vi "Speed Control 1 - Just before second motor.vi"(11 "queue in":refnum<queue>) -> ()   [LabVIEW 2014]
uses:
  controls/UI Data.ctl
  controls/Control ConfigurationSam.ctl
  controls/EncoderController.ctl
  <vilib>/Platform/TimedLoop/XDataNode/timing_clust.ctl
  <vilib>/Platform/TimedLoop/XDataNode/nitl_modes.ctl
  <vilib>/Platform/TimedLoop/XDataNode/wakeup.ctl
  controls/Control StateSam.ctl
  <vilib>/Platform/TimedLoop/XDataNode/loadnilvce.vi
  <vilib>/addons/control/pid/pid.llb/PID (DBL).vi
  <vilib>/addons/control/pid/pid.llb/PID Percentage to EGU (DBL).vi
  <vilib>/platform/TimedLoop/XDataNode/XDataNode.xnode
  <vilib>/addons/control/pid/NI_PID_pid.lvlib
  <vilib>/Platform/TimedLoop/XDataNode/XDNodeRunTimeDep.lvlib
panel:
  out "Velocity4 RPM":dbl
  out "Motor1Output":dbl
  out "Velocity1 RPM":dbl
  # "0.8, 0. 0 is stable but theres a large offset\nsystem is slow to settle, increase Ti"
  # "Kp=2.04, Ti=0.15, Td=0.0375"
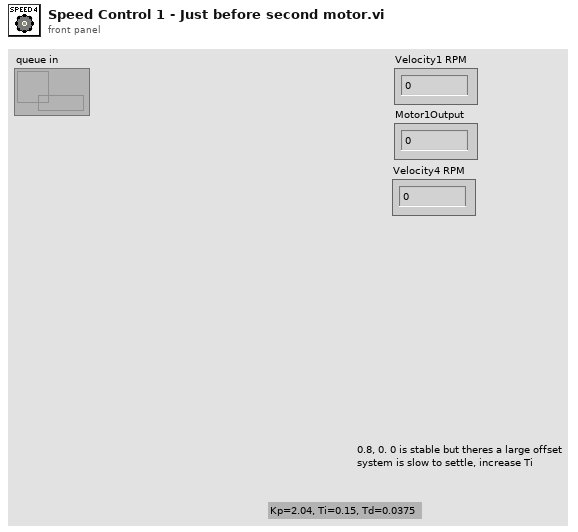
[diagram p1: front panel]
types:
  T1 = typedef "Control ConfigurationSam.ctl" = cluster{"PID Gains":cluster{"proportional gain (Kc)":dbl, "integral gain (Kc*Ts/Ti)":dbl, "derivative gain (Kc*Td/Ts)":dbl}, "Output Range":cluster{"output high":dbl, "output low":dbl}}
  T2 = cluster{bool, "Tick Count(uSec)":u32, "Counter Value":i32, "x-y":i32}
  T3 = typedef "XDNodeRunTimeDep.lvlib/timing_clust.ctl" = cluster{"Expected End [f-1]":u64, "Actual End [f-1]":u64, "Finished Late? [f-1]":bool, "Expected End [i-1]":u64, "Actual End [i-1]":u64, "Finished Late? [i-1]":bool, "Expected Start [i]":u64, "Actual Start [i]":u64, "Expected Start [f]":u64, "Actual Start [f]":u64, "Source Name":string, "Structure Name":string, "Period":i64, "Deadline":i64, "Offset":i64, "Start":i64, "Priority":i32, "Timeout":i32, "Mode":T4, "Wakeup Reason":T5, "Error":errorcluster, "Source Type":string, "Secondary Source Type":string, "Global End Time":u64, "Global Start Time":u64, "Frame Duration":u64, "Iteration Duration":u64, "Assigned CPU":i32, "I/O Scan Engine Mode":u32}
  T4 = typedef "XDNodeRunTimeDep.lvlib/nitl_modes.ctl" = enum32{"No Change", "Process missed periods, maintain original phase", "Discard missed periods, maintain original phase", "Process missed periods, ignore original phase", "Discard missed periods, ignore original phase"}
  T5 = typedef "XDNodeRunTimeDep.lvlib/wakeup.ctl" = enum32{"Normal", "Aborted", "Asynchronous wakeup", "Timing source error", "Timed loop error", "Timeout"}
  T6 = typedef "EncoderController.ctl" = cluster{"Sample time (uS)":u32, "Reset":bool}
  T7 = typedef "EncoderIndicator.ctl" = cluster{"Position":dbl, "Velocity RPM":dbl, "Velocity RPS":dbl}
  T8 = cluster{"proportional gain (Kc)":dbl, "integral gain (Kc*Ts/Ti)":dbl, "derivative gain (Kc*Td/Ts)":dbl}
  T9 = cluster{"proportional gain (Kc)":dbl, "integral gain (Kc*Ts/Ti)":dbl, "derivative gain (Kc*Td/Ts)":dbl}[]
  T10 = typedef "Control StateSam.ctl" = enum16{"", "Control State (PID)", "Safe State"}
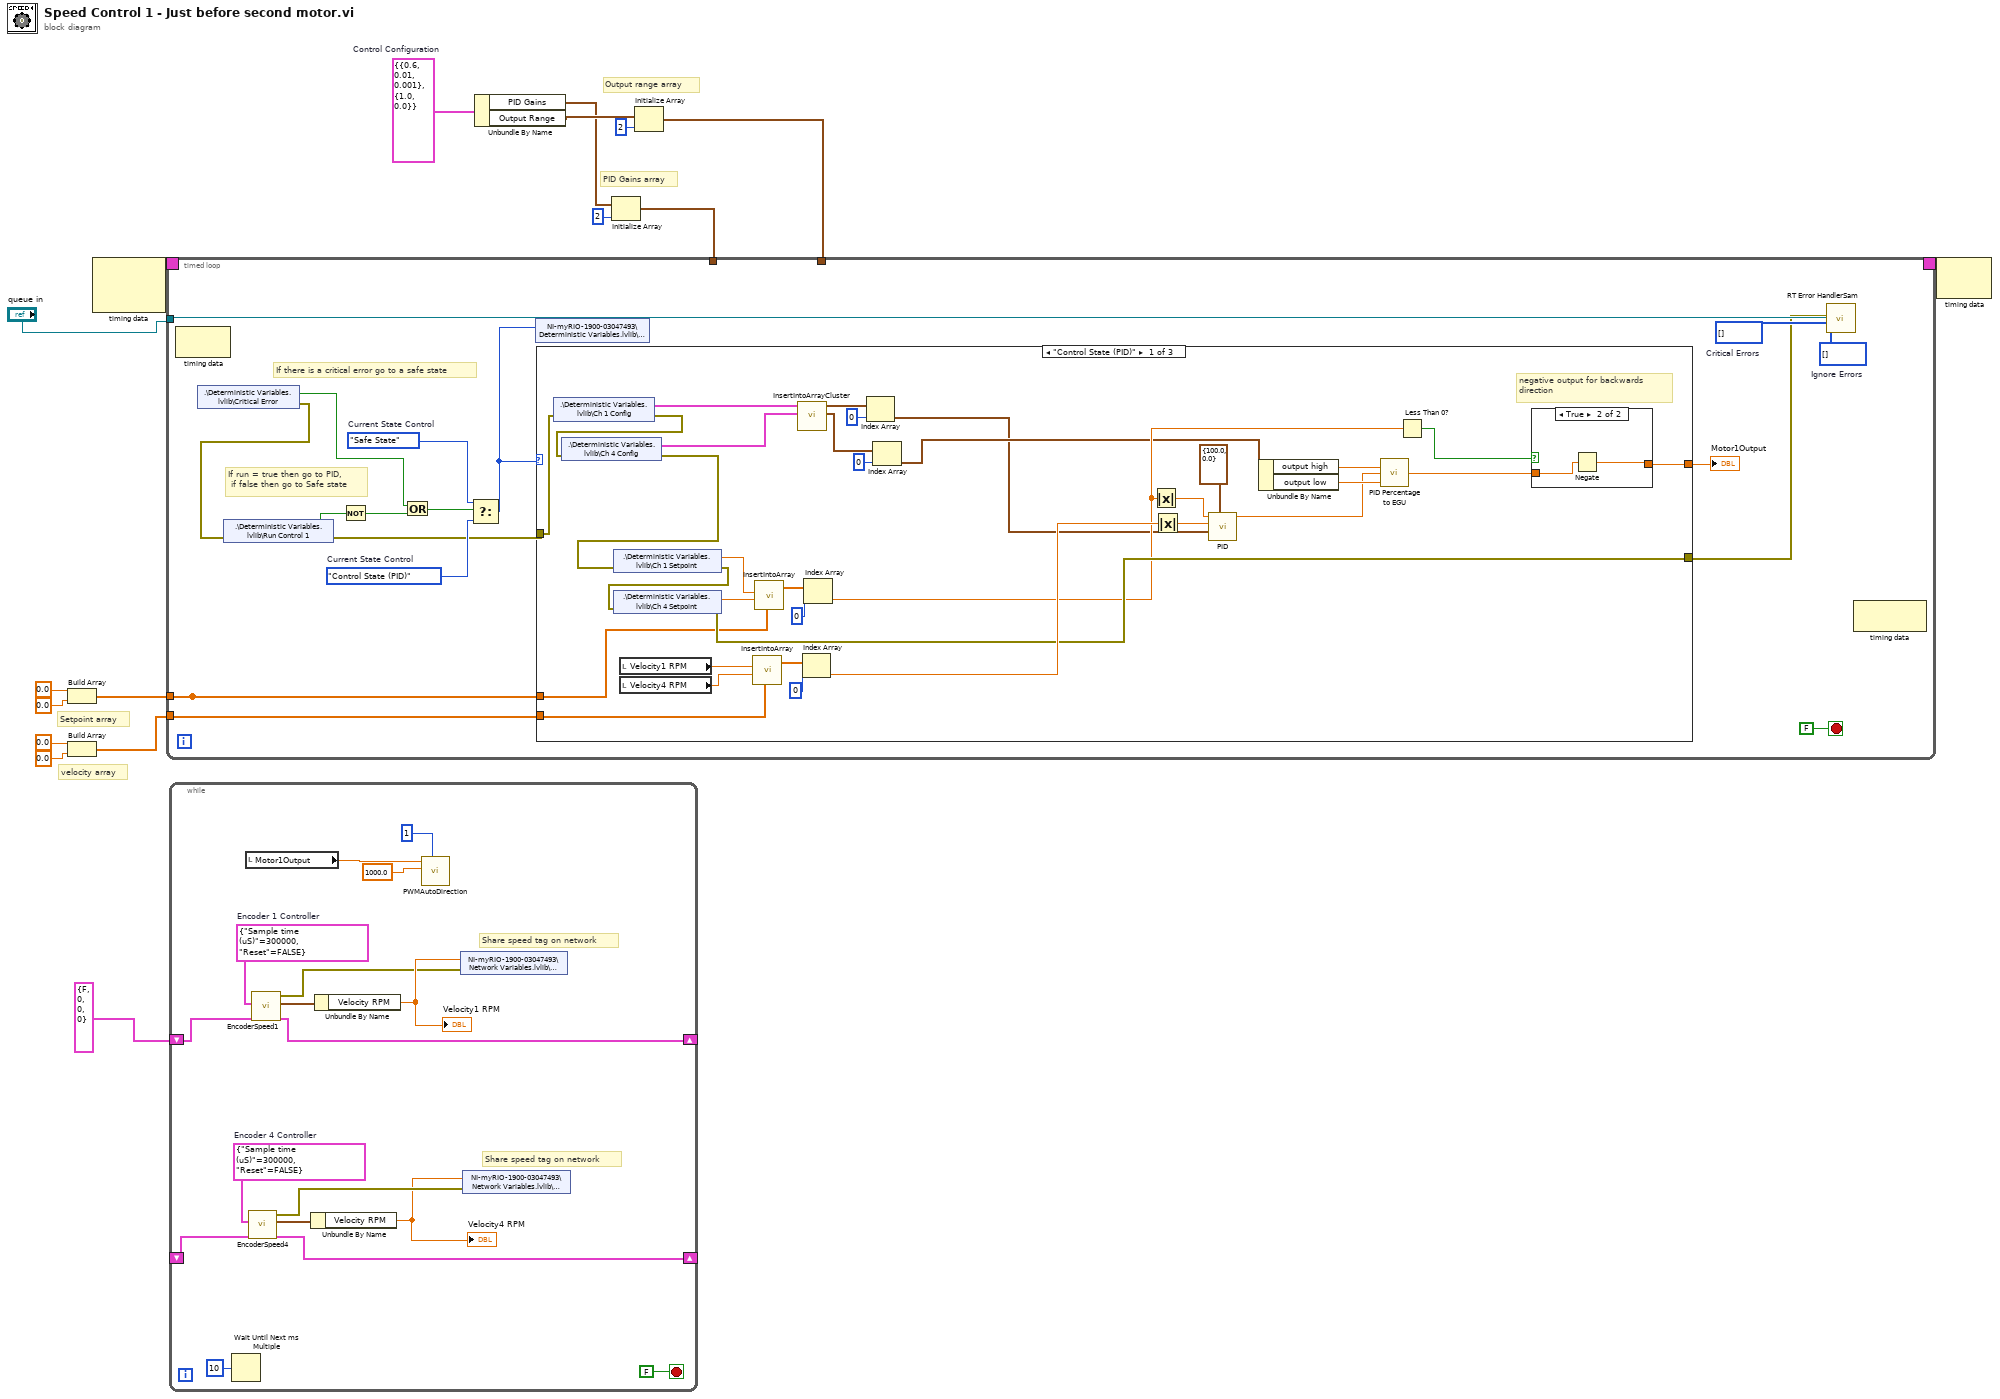
[diagram p0: block diagram]
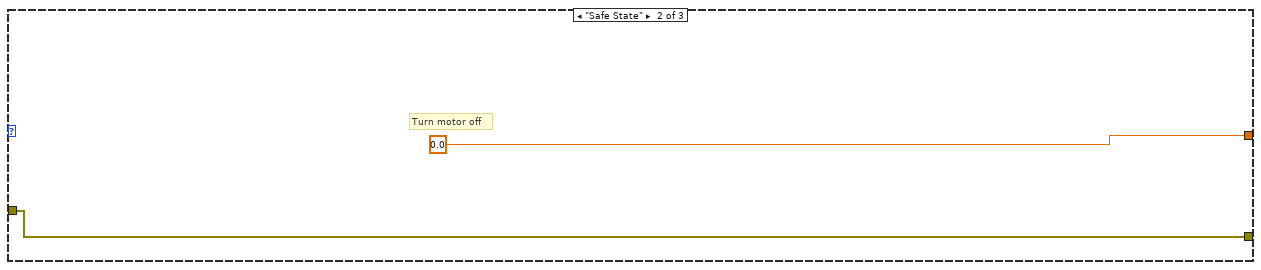
[diagram p3: hidden frame]
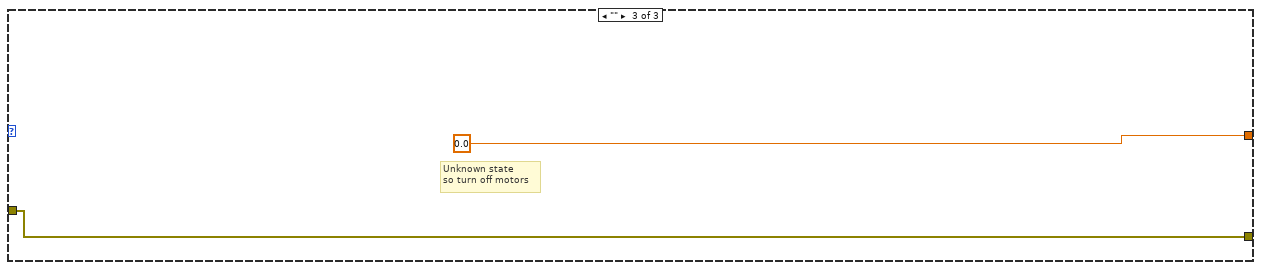
[diagram p4: hidden frame]
diagram:
  w10 = T1 {"PID Gains"={"proportional gain (Kc)"=0.6, "integral gain (Kc*Ts/Ti)"=0.01, "derivative gain (Kc*Td/Ts)"=0.001}, "Output Range"={"output high"=1.0, "output low"=0.0}}  # Control Configuration
  # "Output range array"
  # "velocity array"
  # "PID Gains array"
  # "Setpoint array"
  n1 = Build Array(0.0, 0.0) -> (w4:dbl[])
  n2 = Build Array(0.0, 0.0) -> (w3:dbl[])
  n3 = node-c288() -> (w17:T3)  [unwired: 2 in]
  n4 = while {
    shift-right: [w29] -> _
    shift-left: T2 {FALSE, "Tick Count(uSec)"=0, "Counter Value"=0, "x-y"=0} ("Cluster out") -> [w30]
    shift-right: [w19] -> _
    shift-left: _ -> [w20]
    stop <- FALSE stop-if-true
    w21 = T6 {"Sample time (uS)"=300000, "Reset"=FALSE}  # Encoder 4 Controller
    w34 = T6 {"Sample time (uS)"=300000, "Reset"=FALSE}  # Encoder 1 Controller
    # "Share speed tag on network"
    # "Share speed tag on network"
    n5 = Wait Until Next ms Multiple(millisecond multiple=u32 10) -> ()  [unwired: 1 out]
    n6 = local read "Motor1Output"() -> (w26:dbl)
    n7 = call "EncoderSpeed4.vi"("Cluster in"=w20, "Encoder 4 Controller"=w21) -> ("Cluster out"=w19:T2, "Encoder 4 Indicator"=w22:T7, "error out"=w23:errorcluster)  [unwired: 7 in]
    n8 = call "EncoderSpeed1.vi"("Cluster in"=w30, "Encoder 1 Controller"=w34) -> ("Cluster out"=w29:T2, "Encoder 1 Indicator"=w33:T7, "error out"=w31:errorcluster)  [unwired: 7 in]
    n9 = Unbundle By Name(w22) -> ("Velocity RPM"=w18:dbl)
    "Velocity4 RPM" <- w18
    n10 = Unbundle By Name(w33) -> ("Velocity RPM"=w32:dbl)
    "Velocity1 RPM" <- w32
    n11 = call "PWMAutoDirection.vi"("Motor Select"=i8 1, "PWM Frequency"=1000.0, "DutyCycle"=w26) -> ()  [unwired: 8 in, 1 out]
    n12 = shared-variable "NI-myRIO-1900-03047493\\Network Variables.lvlib\\SpeedMotor1"(w32, error in=w31) -> ()  [unwired: 1 out]
    n13 = shared-variable "NI-myRIO-1900-03047493\\Network Variables.lvlib\\SpeedMotor4"(w18, error in=w23) -> ()  [unwired: 1 out]
  }
  n14 = Unbundle By Name(w10) -> ("PID Gains"=w11:T8, "Output Range"=w13:cluster{"output high":dbl, "output low":dbl})
  n15 = Initialize Array(w11, 2 ("dimension size")) -> (w2:T9)
  n16 = Initialize Array(w13, 2 ("dimension size")) -> (w1:cluster{"output high":dbl, "output low":dbl}[])
  n17 = timed-loop {
    timing: w17 -> [_]
    timing-out: [_] -> w16
    tunnel: "queue in" -> [w39]
    tunnel: [w35] -> _
    tunnel: w4 -> [w35]
    tunnel: w3 -> [w36]
    tunnel: w2 -> [_]
    tunnel: w1 -> [_]
    stop <- FALSE stop-if-true
    w40 = i32[] []  # Critical Errors
    w41 = i32[] []  # Ignore Errors
    w48 = Control_StateSam."Control State (PID)"  # Current State Control
    w49 = Control_StateSam."Safe State"  # Current State Control
    # "If there is a critical error go to a safe state"
    # "If run = true then go to PID,\n if false then go to Safe state"
    n18 = node-c288() -> ()  [unwired: 1 in, 1 out]
    n19 = shared-variable ".\\Deterministic Variables.lvlib\\Critical Error"() -> (w45:bool, error out=w43:errorcluster)  [unwired: 1 in]
    n20 = shared-variable ".\\Deterministic Variables.lvlib\\Run Control 1"(error in=w43) -> (w50:bool, error out=w42:errorcluster)
    n21 = Not(x=w50) -> (.not. x?=w46:bool)
    n22 = Or(x=w45, y=w46) -> (x .or. y?=w44:bool)
    n23 = Select(t=w49, s=w44, f=w48) -> (s? t:f=w47:T10)
    n24 = shared-variable "NI-myRIO-1900-03047493\\Deterministic Variables.lvlib\\Control State 1"(w47) -> ()  [unwired: 1 in, 1 out]
    n25 = case shown="\"Control State (PID)\"" w47 {
      tunnel: [w78 0.0 ("output (EGU)") 0.0 ("output (EGU)")] -> w38
      tunnel: w42 -> [w81 w89 w91]
      tunnel: [w68 w89 w91] -> w37
      tunnel: w36 -> [w73 _ _]
      tunnel: w35 -> [w63 _ _]
      frame "Control State (PID)" {
        # "negative output for backwards \ndirection"
        n26 = shared-variable ".\\Deterministic Variables.lvlib\\Ch 1 Config"(error in=w81) -> (w59:T1, error out=w61:errorcluster)
        n27 = shared-variable ".\\Deterministic Variables.lvlib\\Ch 4 Config"(error in=w61) -> (w58:T1, error out=w60:errorcluster)
        n28 = shared-variable ".\\Deterministic Variables.lvlib\\Ch 1 Setpoint"(error in=w60) -> (w65:dbl, error out=w69:errorcluster)
        n29 = shared-variable ".\\Deterministic Variables.lvlib\\Ch 4 Setpoint"(error in=w69) -> (w64:dbl, error out=w68:errorcluster)
        n30 = local read "Velocity1 RPM"() -> (w75:dbl)
        n31 = local read "Velocity4 RPM"() -> (w74:dbl)
        n32 = call "InsertIntoArray.vi"("input array"=w73, "new element 1"=w74, "new element 0"=w75) -> ("output array"=w72:dbl[])  [unwired: 8 in]
        n33 = call "InsertIntoArray.vi"("input array"=w63, "new element 1"=w64, "new element 0"=w65) -> ("output array"=w66:dbl[])  [unwired: 8 in]
        n34 = call "InsertIntoArrayCluster.vi"("CH2"=w58, "CH1"=w59) -> ("Output Range array"=w54:cluster{"output high":dbl, "output low":dbl}[], "PID Gains array"=w57:T9)  [unwired: 8 in]
        n35 = Index Array(array=w72, index=0) -> (element=w70:dbl)
        n36 = Index Array(array=w66, index=0) -> (element=w62:dbl)
        n37 = Index Array(array=w57, index=0) -> (element=w52:T8)
        n38 = Index Array(array=w54, index=0) -> (element=w53:cluster{"output high":dbl, "output low":dbl})
        n39 = Absolute Value(x=w62) -> (abs(x)=w77:dbl)
        n40 = Absolute Value(x=w70) -> (abs(x)=w76:dbl)
        n41 = call-poly <vilib>:"PID.vi"("output range"=cluster{"output high":dbl, "output low":dbl} {"output high"=100.0, "output low"=0.0}, "PID gains"=w52, "process variable"=w76, "setpoint"=w77) -> ("output"=w83:dbl)  [unwired: 6 in, 1 out]
        n42 = Unbundle By Name(w53) -> ("output high"=w85:dbl, "output low"=w84:dbl)
        n43 = call-poly <vilib>:"PID Percentage to EGU.vi"("minimum (EGU)"=w84, "% span"=w83, "maximum (EGU)"=w85) -> ("output (EGU)"=w79:dbl)  [unwired: 1 in]
        n44 = Less Than 0?(x=w62) -> (x < 0?=w80:bool)
        n45 = case shown="True" w80 {
          tunnel: w79 -> [w86 w88]
          tunnel: [w86 w87] -> w78
          frame False {
          }
          frame True {
            n46 = Negate(x=w88) -> (-x=w87:dbl)
          }
        }
      }
      frame "Safe State" {
        # "Turn motor off"
      }
      frame "" {
        # "Unknown state\nso turn off motors"
      }
    }
    "Motor1Output" <- w38
    n47 = call "RT Error HandlerSam.vi"("Ignore Errors"=w41, "Critical Errors"=w40, "error to process"=w37, "queue in"=w39) -> ()  [unwired: 7 in, 1 out]
    n48 = node-c288() -> ()  [unwired: 1 in, 1 out]
  }
  n49 = node-c288(w16) -> ()  [unwired: 1 out]
